vi "WarpPerspectiveARGB.vi"(4 "Border Colour (Default: Black)":T2={"Alpha"=255, "RGB"=0}, 5 "Boarder Type (Default: DEFAULT)":T3=enum."DEFAULT", 6 "Required Destination Size":T5, 7 "Interpolation Mode (Default: CUBIC)":T4=enum."CUBIC", 8 "error in (no error)":errorcluster, 9 "3x3 Warp Matrix":T1, 10 "ARGB Destination Image":refnum<data-value>, 11 "ARGB Source Image":refnum<data-value>) -> (0 "error out":errorcluster, 3 "ARGB  Destination Image (duplicate)":refnum<data-value>)   [LabVIEW 2020, in "g_ar_toolkit.image.lvlib"]
uses:
  g_ar_toolkit.image.lvlib
  g_ar_toolkit.common/Image Size (Integer).ctl
  Interpolation Mode.ctl
  Border Type.ctl
  ARGB Colour.ctl
  <vilib>/Analysis/Matrix/Datatypes/RealMatrix.ctl
  2e2371c9-0103-42e0-a64c-538b92d2b12b.vi/0c263cf4-9042-4d44-b92e-dafa676e1650.vi
  <vilib>/Utility/error.llb/Error Cluster From Error Code.vi
  2e2371c9-0103-42e0-a64c-538b92d2b12b.vi
  g_ar_toolkit.common/g_ar_toolkit_common.lvlib
  <vilib>/Analysis/Matrix/NI_Matrix.lvlib
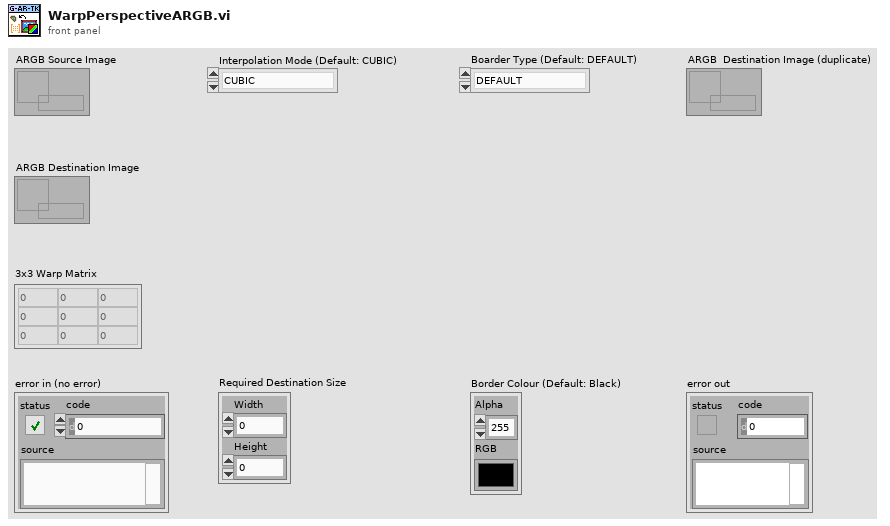
[diagram p1: front panel]
types:
  T1 = typedef "NI_Matrix.lvlib/RealMatrix.ctl" = dbl[][]
  T2 = typedef "g_ar_toolkit.image.lvlib/ARGB Colour.ctl" = cluster{"Alpha":u8, "RGB":u32}
  T3 = typedef "g_ar_toolkit.image.lvlib/Border Type.ctl" = enum8{"CONSTANT", "REPLICATE", "REFLECT", "WRAP", "TRANSPARENT", "DEFAULT", "ISOLATED"}
  T4 = typedef "g_ar_toolkit.image.lvlib/Interpolation Mode.ctl" = enum8{"NEAREST", "LINEAR", "CUBIC", "AREA", "LANCZOS", "LINEAR_EXACT", "NEAREST_EXACT", "MAX"}
  T5 = typedef "g_ar_toolkit_common.lvlib/Image Size (Integer).ctl" = cluster{"Width":u16, "Height":u16}
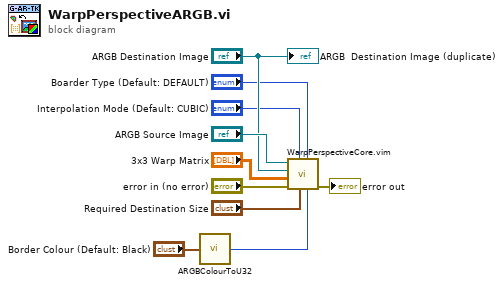
[diagram p0: block diagram]
diagram:
  n1 = call "ARGBColourToU32.vi"("ARGB Colour"="Border Colour (Default: Black)") -> ("U32 Colour"=w1:u32)
  n2 = call "WarpPerspectiveCore.vim"("Border Colour"=w1, "Boarder Type"="Boarder Type (Default: DEFAULT)", "Destination Size"="Required Destination Size", "Interpolation Mode"="Interpolation Mode (Default: CUBIC)", "error in (no error)"="error in (no error)", "Homography"="3x3 Warp Matrix", "Dst"="ARGB Destination Image", "Src"="ARGB Source Image") -> ("error out"=→"error out":errorcluster)  [unwired: 3 in]
  "ARGB  Destination Image (duplicate)" <- "ARGB Destination Image"
